vi "温度曲线显示.vi"() -> ()   [LabVIEW 2016, in "斯坦道总氮.lvlib"]
panel:
  out "显示值":string
  in  "历史曲线":bool
  in  "单选按钮":enum32{"消解温度曲线", "注射器温度曲线"}(radio)
  in  "关闭":bool
  out "波形图":dbl[](graph)
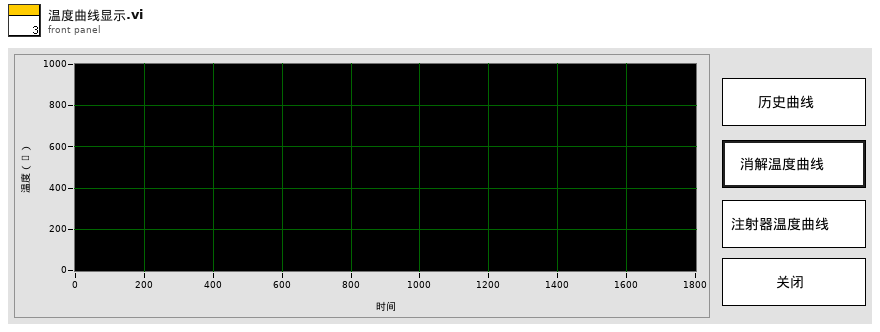
[diagram p1: front panel]
types:
  T1 = typedef "LVPoint32TypeDef.ctl" = cluster{"Horizontal":i32, "Vertical":i32}
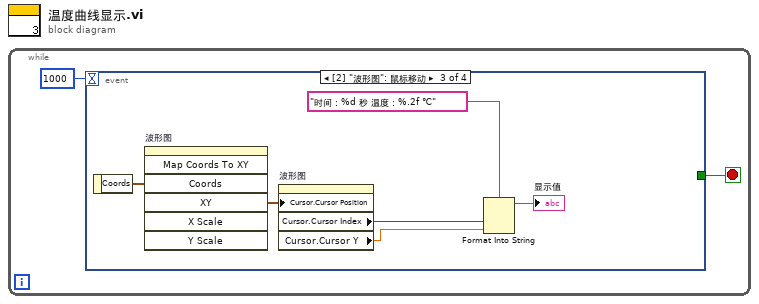
[diagram p0: block diagram]
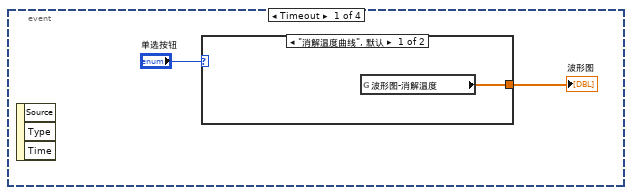
[diagram p2: hidden frame]
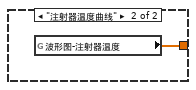
[diagram p3: hidden frame]
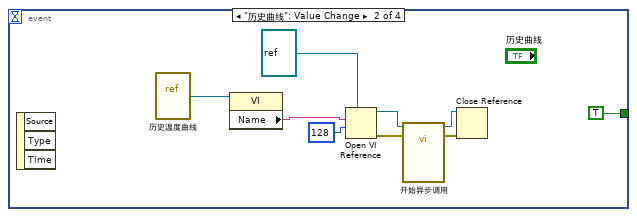
[diagram p4: hidden frame]
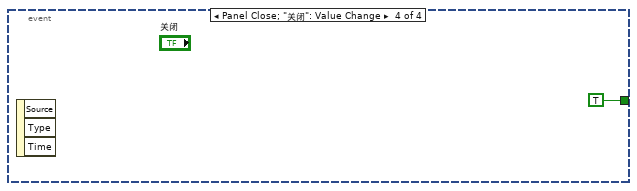
[diagram p5: hidden frame]
diagram:
  n1 = while {
    stop <- w2 stop-if-true
    n2 = event shown="[2] \"波形图\": 鼠标移动" {
      selector: _ -> [_ _ _ _]
      dyn-events: _ -> [_ _ _ _]
      timeout: 1000 -> [_ _ _ _]
      tunnel: [_ TRUE _ TRUE] -> w2
      event Timeout {
        n3 = event-data() -> ()  [unwired: 1 in, 3 out]
        n4 = case shown="\"消解温度曲线\", 默认" "单选按钮" {
          tunnel: [w5 w6] -> w3
          frame "消解温度曲线", Default {
            n5 = global read "VAR总磷总氮全局变量.vi" "波形图-消解温度"() -> (w5:dbl[])
          }
          frame "注射器温度曲线" {
            n6 = global read "VAR总磷总氮全局变量.vi" "波形图-注射器温度"() -> (w6:dbl[])
          }
        }
        "波形图" <- w3
      }
      event "历史曲线": Value Change {
        n7 = event-data() -> ()  [unwired: 1 in, 3 out]
        n8 = vi-ref "历史温度曲线.vi"() -> (w7:refnum<vi>)
        n9 = property class="VI"(reference=w7) -> ("Name"=w8:string)  [unwired: 1 in, 2 out]
        n10 = Open VI Reference(type specifier VI Refnum (for type only)=refnum<vi> refnum, vi path=w8, options=128 ("选项")) -> (vi reference=w11:refnum<vi>, error out=w12:errorcluster)  [unwired: 3 in]
        n11 = call-by-ref "开始异步调用"(reference=w11, error in=w12) -> (reference out=w13:refnum<vi>, error out=w14:errorcluster)  [unwired: 12 in]
        n12 = Close Reference(reference=w13, error in (no error)=w14) -> ()  [unwired: 1 out]
      }
      event "波形图": Mouse Move {
        n13 = event-data() -> ("Coords"=w21:T1)  [unwired: 1 in]
        n14 = invoke on="波形图" class="WFGraph (严格)" method="Map Coords To XY"("Coords"=w21) -> ("XY"=w20:cluster{"X":dbl, "Y":dbl})  [unwired: 6 in, 6 out]
        n15 = property on="波形图" class="WFGraph (严格)"("Cursor.Cursor Position"=w20) -> ("Cursor.Cursor Index"=w17:i32, "Cursor.Cursor Y"=w16:dbl)  [unwired: 2 in, 2 out]
        n16 = Format Into String(format string="时间：%d 秒 温度：%.2f ℃" ("格式字符串"), w17, w16) -> (resulting string=→"显示值":string)  [unwired: 2 in, 1 out]
      }
      event Panel Close; "关闭": Value Change {
        n17 = event-data() -> ()  [unwired: 1 in, 3 out]
      }
    }
  }
